vi "Validate Selected Client Names.vi"(8 "error in (no error)":errorcluster, 10 "project ref":refnum<vi>, 11 "multicolumnListbox in":refnum<vi>) -> (0 "error out":errorcluster, 1 "selected client names":string[](array[string]), 2 "selected measurement indices":i32[](array[numeric]), 3 "multicolumnListbox out":refnum<vi>, 4 "warning?":bool)   [LabVIEW 2021, in "MeasurementClient Editor.lvlib"]
uses:
  MeasurementClient Editor.lvlib
  <vilib>/Utility/miscctls.llb/LVRowAndColumnTypeDef.ctl
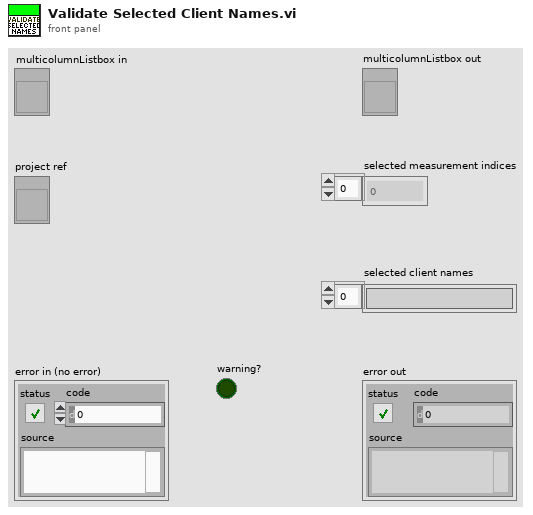
[diagram p1: front panel]
types:
  T1 = typedef "LVRowAndColumnTypeDef.ctl" = cluster{"Row":i32, "Column":i32}
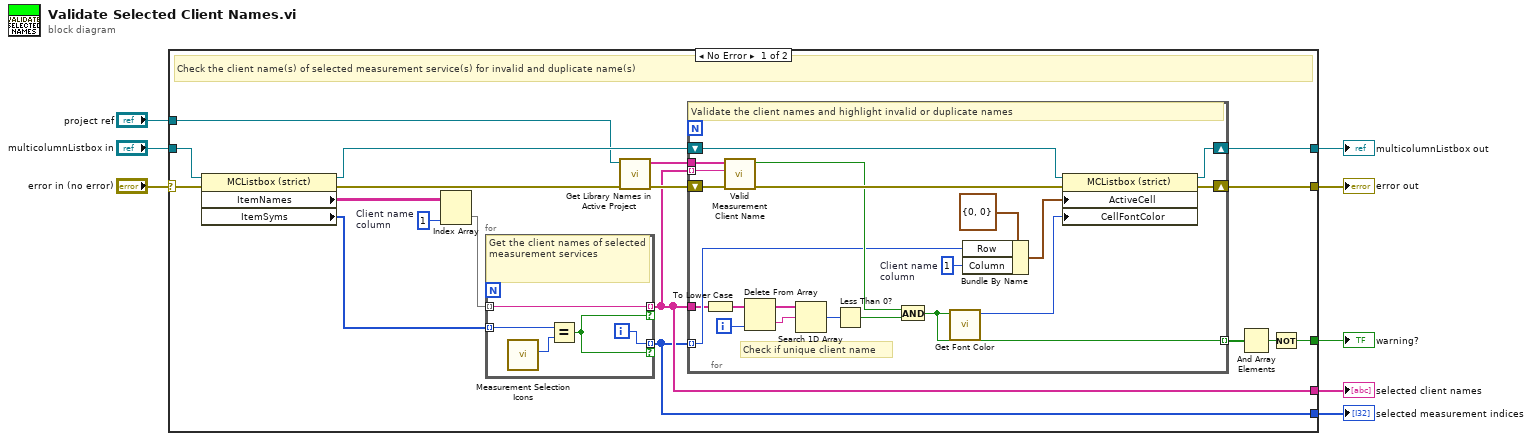
[diagram p0: block diagram]
diagram:
  n1 = case shown="No Error" "error in (no error)" {
    selector: "error in (no error)" -> [w25 w54]
    tunnel: "multicolumnListbox in" -> [w26 w53]
    tunnel: [w22 w54] -> w6
    tunnel: [w21 w53] -> w5
    tunnel: [w14 _] -> w4
    tunnel: "project ref" -> [w19 _]
    tunnel: [w10 _] -> w2
    tunnel: [w9 _] -> w1
    frame No Error {
      w24 = 1  # Client name column
      # "Check the client name(s) of selected measurement service(s) for invalid and duplicate name(s)"
      n2 = property class="MCListbox (strict)"(reference=w26, error in=w25) -> (reference out=w23:refnum<vi>, error out=w17:errorcluster, "ItemNames"=w16:string[][], "ItemSyms"=w11:i32[])
      n3 = Index Array(array=w16, index (col)=w24) -> (element=w12:string[])  [unwired: 1 in]
      n4 = for {
        tunnel: w12 -> [w50] mode=indexing
        tunnel: w11 -> [w52] mode=indexing
        tunnel: [w50] -> w10 mode=indexing if=w48
        tunnel: [w49] -> w9 mode=indexing if=w48
        i -> [w49]
        # "Get the client names of selected measurement services"
        n5 = call "Measurement Selection Icons.vi"() -> ("Checked"=w51:i32)  [unwired: 10 in, 1 out]
        n6 = Equal?(x=w52, y=w51) -> (x = y?=w48:bool)
      }
      n7 = call "Get Library Names in Active Project.vi"("error in (no error)"=w17, "project ref"=w19) -> ("error out"=w20:errorcluster, "library names"=w18:string[])  [unwired: 8 in]
      n8 = for {
        shift-right: [w41] -> w22
        shift-left: w20 -> [w47]
        shift-right: [w40] -> w21
        shift-left: w23 -> [w45]
        tunnel: w10 -> [w31]
        tunnel: w18 -> [w33]
        tunnel: w10 -> [w27] mode=indexing
        tunnel: w9 -> [w32] mode=indexing
        tunnel: [w28] -> w13 mode=indexing
        i -> [w30]
        w42 = 1  # Client name column
        # "Check if unique client name"
        # "Validate the client names and highlight invalid or duplicate names"
        n9 = To Lower Case(string=w31) -> (all lower case string=w34:string[])
        n10 = call "Valid Measurement Client Name.vi"("error in"=w47, "requested client name"=w27, "library names"=w33) -> ("error out"=w46:errorcluster, "valid name?"=w35:bool)  [unwired: 7 in]
        n11 = Delete From Array(array=w34, index=w30) -> (deleted portion=w38:string, array with subset deleted=w39:string[])  [unwired: 1 in]
        n12 = Search 1D Array(1D array=w39, element=w38) -> (index of element=w37:i32)  [unwired: 1 in]
        n13 = Less Than 0?(x=w37) -> (x < 0?=w36:bool)
        n14 = And(x=w35, y=w36) -> (x .and. y?=w28:bool)
        n15 = call "Get Font Color.vi"("valid?"=w28) -> ("font colour"=w29:u32)  [unwired: 10 in]
        n16 = Bundle By Name(cluster=T1 {"Row"=0, "Column"=0} ("Active Cell:Active Cell"), "Row"=w32, "Column"=w42) -> (w43:T1)
        n17 = property class="MCListbox (strict)"(reference=w45, error in=w46, "ActiveCell"=w43, "CellFontColor"=w29) -> (reference out=w40:refnum<vi>, error out=w41:errorcluster)
      }
      n18 = And Array Elements(Boolean array=w13) -> (logical AND=w15:bool)
      n19 = Not(x=w15) -> (.not. x?=w14:bool)
    }
    frame Error {
      # "Pass"
    }
  }
  "error out" <- w6
  "multicolumnListbox out" <- w5
  "warning?" <- w4
  "selected measurement indices" <- w1
  "selected client names" <- w2
